vi "Safe Stop.vi"() -> (0 "Time has Elapsed":bool)   [LabVIEW 2013]
uses:
  Robot Global Data.vi
panel:
  out "sound":bool
  in  "Evil angle":dbl=95.0
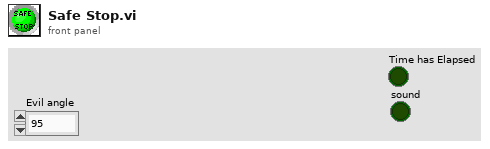
[diagram p1: front panel]
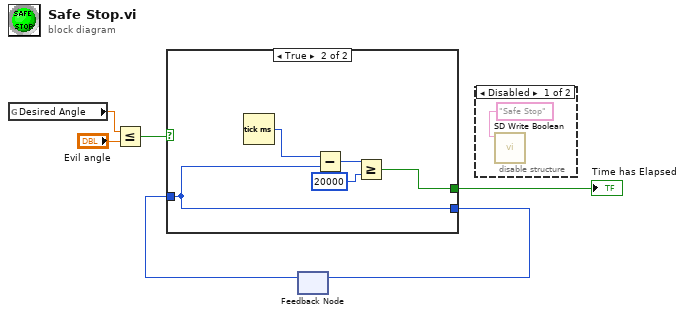
[diagram p0: block diagram]
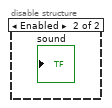
[diagram p2: hidden frame]
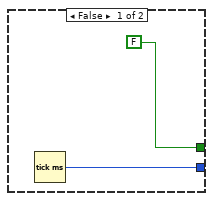
[diagram p3: hidden frame]
diagram:
  n1 = global read "Robot Global Data.vi" "Desired Angle"() -> (w3:dbl)
  n2 = Less Or Equal?(x=w3, y="Evil angle") -> (x <= y?=w5:bool)
  n3 = feedback #1() -> (w1:u32)  [unwired: 1 in]
  n4 = case shown="True" w5 {
    tunnel: [FALSE w10] -> w4
    tunnel: [w8 w9] -> w2
    tunnel: w1 -> [_ w9]
    frame False {
      n5 = Tick Count (ms)() -> (millisecond timer value=w8:u32)
    }
    frame True {
      n6 = Tick Count (ms)() -> (millisecond timer value=w13:u32)
      n7 = Subtract(x=w13, y=w9) -> (x-y=w12:u32)
      n8 = Greater Or Equal?(x=w12, y=u32 20000) -> (x >= y?=w10:bool)
    }
  }
  "Time has Elapsed" <- w4
  n9 = feedback-in #1(w2) -> ()
  n10 = disable-structure shown="Disabled" {
    frame Disabled {
      n11 = call <vilib>:"SD Write Boolean.vi"("Name"="Safe Stop") -> ()  [unwired: 9 in, 2 out]
    }
    frame Enabled {
    }
  }
